vi "Finish.vi"   [LabVIEW 2014]
doc: "This VI is called just before exiting. It is expected to close I/O refnum, save collected data, etc."
uses:
  <vilib>/Rock Robotics/WPI/Joystick/WPI_JoystickGetSetRefNum.vi
  <vilib>/Rock Robotics/WPI/RobotDrive/WPI_RobotDriveGetSetRefNum.vi
  <vilib>/Rock Robotics/WPI/Compressor/WPI_CompressorGetSetRefNum.vi
types:
  T1 = typedef "WPI_MotorControlDeviceRef.ctl" = cluster{"DeviceStatus":errorcluster, "Type":T2, "PWM":cluster{"Controller":T3, "PWM Channel":T4, "DeadBand":T5}, "CAN":cluster{"Device Number":u8, "Control Mode":T6, "Semaphore":T7, "Max Vout":dbl, "TalonSRX Control Mode":T8}, "Invert":bool, "TransformRef":T9, "InvTransformRef":T9}
  T2 = typedef "WPI_MotorControlType.ctl" = enum16{"PWM", "CAN", "CANTalonSRX"}
  T3 = typedef "FPGA_TypedefDigitalModule.ctl" = enum16{"Controller 1"}
  T4 = typedef "FPGA_DIOPWMChannel.ctl" = enum8{"PWM 0", "PWM 1", "PWM 2", "PWM 3", "PWM 4", "PWM 5", "PWM 6", "PWM 7", "PWM 8", "PWM 9", "PWM MXP 0", "PWM MXP 1", "PWM MXP 2", "PWM MXP 3", "PWM MXP 4", "PWM MXP 5", "PWM MXP 6", "PWM MXP 7", "PWM MXP 8", "PWM MXP 9", "Invalid"}
  T5 = typedef "WPI_PWMDeadband.ctl" = cluster{"Name":string, "maxPositivePwm":i32, "minPositivePwm":i32, "centerPwm":i32, "maxNegativePwm":i32, "minNegativePwm":i32, "angularRange":u16}
  T6 = typedef "WPI_CANJaguar_ControlMode.ctl" = enum8{"Percent VBus", "Current", "Speed", "Position", "Voltage"}
  T7 = typedef "Semaphore RefNum" = refnum<k1>
  T8 = typedef "WPI_CANTalonSRX_APIControlMode.ctl" = enum8{"Percent VBus", "Speed", "Position", "Slave", "Unchanged / Invalid"}
  T9 = typedef "WPI_PWMTransform_ConPane.ctl" = refnum<vi>
  T10 = typedef "WPI_JoystickDevRef.ctl" = cluster{"Device":T11}
  T11 = typedef "WPI_JoystickDeviceEnum.ctl" = enum16{"USB 0", "USB 1", "USB 2", "USB 3", "USB 4", "USB 5"}
  T12 = typedef "WPI_RobotDriveDevRef.ctl" = cluster{"DevStatus":errorcluster, "Motors[]":T1[], "Square Inputs":bool, "Max Output":dbl}
  T13 = typedef "WPI_PotentiometerDevRef.ctl" = cluster{"DevStatus":errorcluster, "Controller":T14, "Analog Channel":T15, "Invert Output":bool}
  T14 = typedef "FPGA_TypedefAnalogModule.ctl" = enum16{"Controller 1"}
  T15 = typedef "FPGA_AIChannel.ctl" = enum8{"AI 0", "AI 1", "AI 2", "AI 3", "AI MXP 0", "AI MXP 1", "AI MXP 2", "AI MXP 3", "Invalid"}
  T16 = typedef "WPI_SolenoidDevRef.ctl" = cluster{"DevStatus":errorcluster, "Pneumatics Control Module":u8, "Forward Solenoid Channel":T17, "Reverse Solenoid Channel":T17}
  T17 = typedef "WPI_SolenoidChannel.ctl" = enum8{"Solenoid 0", "Solenoid 1", "Solenoid 2", "Solenoid 3", "Solenoid 4", "Solenoid 5", "Solenoid 6", "Solenoid 7", "Invalid"}
  T18 = typedef "WPI_SwitchDevRef.ctl" = cluster{"DevStatus":errorcluster, "DIO Channel":T19, "Controller":T3, "CntIndex":T20, "Normally Closed":bool}
  T19 = typedef "FPGA_DIOChannel.ctl" = enum8{"DIO 0", "DIO 1", "DIO 2", "DIO 3", "DIO 4", "DIO 5", "DIO 6", "DIO 7", "DIO 8", "DIO 9", "DIO MXP 0", "DIO MXP 1", "DIO MXP 2", "DIO MXP 3", "DIO MXP 4", "DIO MXP 5", "DIO MXP 6", "DIO MXP 7", "DIO MXP 8", "DIO MXP 9", "DIO MXP 10", "DIO MXP 11", "DIO MXP 12", "DIO MXP 13", "DIO MXP 14", "DIO MXP 15", "Invalid"}
  T20 = typedef "FPGA_CounterCtrSystemIndex.ctl" = enum8{"Ctr 0", "Ctr 1", "Ctr 2", "Ctr 3", "Ctr 4", "Ctr 5", "Ctr 6", "Ctr 7", "Invalid"}
  T21 = typedef "WPI_CompressorDevRef.ctl" = cluster{"DevStatus":errorcluster, "Pneumatics Control Module":u8}
  T22 = typedef "WPI_EncoderDevRef.ctl" = cluster{"DevStatus":errorcluster, "EncoderIndex":T23, "CounterIndex":T20, "DistancePerCount":dbl, "Decoding Type":T24}
  T23 = typedef "FPGA_EncoderIdx.ctl" = enum8{"Enc 0", "Enc 1", "Enc 2", "Enc 3", "Enc 4", "Enc 5", "Enc 6", "Enc 7", "Invalid"}
  T24 = typedef "WPI_EncoderType.ctl" = enum16{"1x", "2x", "4x"}
  T25 = typedef "WPI_GyroDevRef.ctl" = cluster{"DevStatus":errorcluster, "Analog Module":T14, "Analog Channel":T15, "Offset":dbl, "Gain (VoltsPerDegree/Second)":dbl}
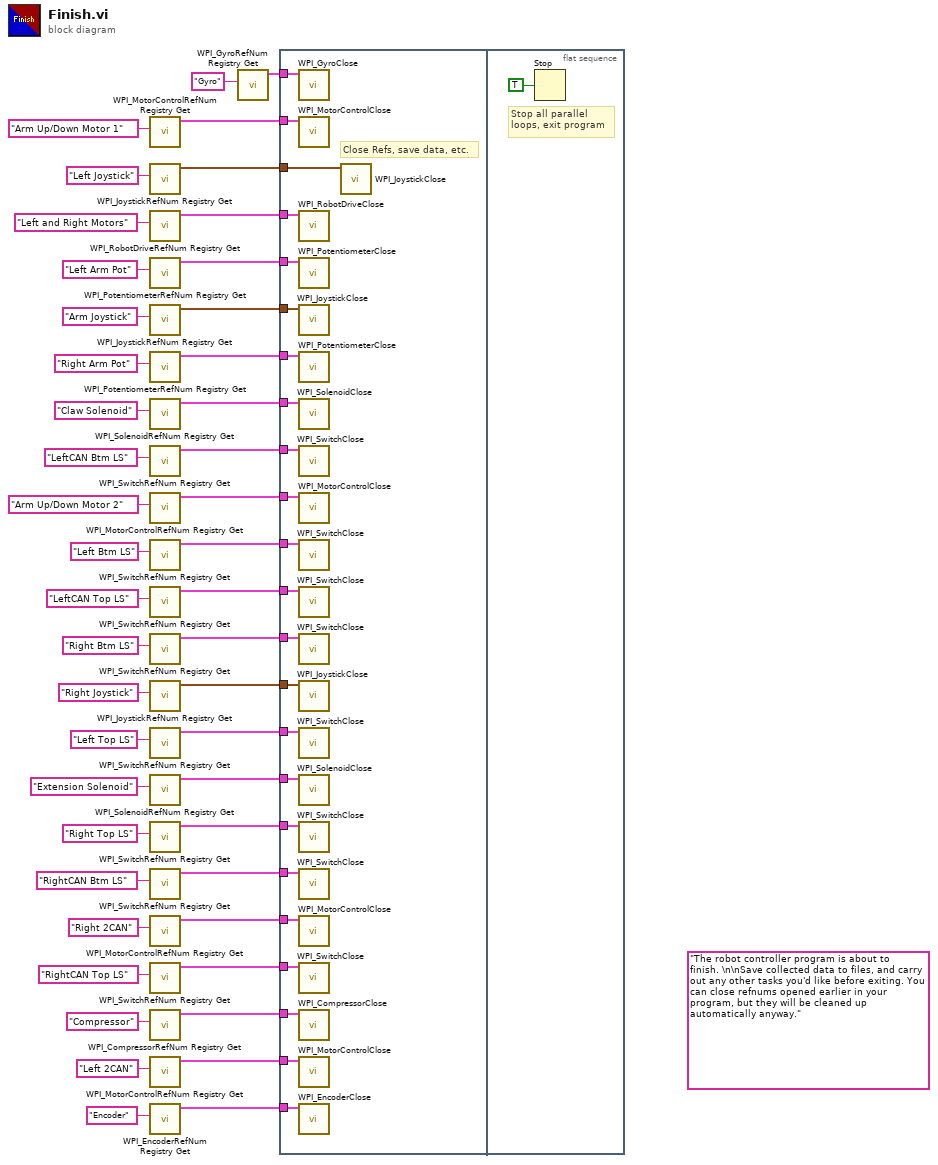
[diagram p0: block diagram]
diagram:
  (unwired) "The robot controller program is about to finish. \n\nSave collected data to files, and carry out any other tasks you'd like before exiting. You can close refnums opened earlier in your program, but they will be cleaned up automatically anyway."
  n1 = call <vilib>:"WPI_MotorControlRefNum Registry Get.vi"("refnum name"="Arm Up/Down Motor 1") -> ("MotorControlDevRef"=w33:T1)  [unwired: 9 in, 1 out]
  n2 = call <vilib>:"WPI_JoystickRefNum Registry Get.vi"("refnum name"="Left Joystick") -> ("JoystickDevRef"=w43:T10)  [unwired: 1 in, 9 out]
  n3 = call <vilib>:"WPI_RobotDriveRefNum Registry Get.vi"("refnum name"="Left and Right Motors") -> ("RobotDriveDevRef"=w44:T12)  [unwired: 1 in, 9 out]
  n4 = call <vilib>:"WPI_PotentiometerRefNum Registry Get.vi"("refnum name"="Left Arm Pot") -> ("PotDevRef"=w13:T13)  [unwired: 9 in, 1 out]
  n5 = call <vilib>:"WPI_JoystickRefNum Registry Get.vi"("refnum name"="Arm Joystick") -> ("JoystickDevRef"=w40:T10)  [unwired: 1 in, 9 out]
  n6 = call <vilib>:"WPI_PotentiometerRefNum Registry Get.vi"("refnum name"="Right Arm Pot") -> ("PotDevRef"=w12:T13)  [unwired: 9 in, 1 out]
  n7 = call <vilib>:"WPI_SolenoidRefNum Registry Get.vi"("refnum name"="Claw Solenoid") -> ("SolenoidDevRef"=w31:T16)  [unwired: 9 in, 1 out]
  n8 = call <vilib>:"WPI_SwitchRefNum Registry Get.vi"("refnum name"="LeftCAN Btm LS") -> ("SwitchDevRef"=w6:T18)  [unwired: 9 in, 1 out]
  n9 = call <vilib>:"WPI_MotorControlRefNum Registry Get.vi"("refnum name"="Arm Up/Down Motor 2") -> ("MotorControlDevRef"=w28:T1)  [unwired: 9 in, 1 out]
  n10 = call <vilib>:"WPI_SwitchRefNum Registry Get.vi"("refnum name"="Left Btm LS") -> ("SwitchDevRef"=w15:T18)  [unwired: 9 in, 1 out]
  n11 = call <vilib>:"WPI_SwitchRefNum Registry Get.vi"("refnum name"="LeftCAN Top LS") -> ("SwitchDevRef"=w5:T18)  [unwired: 9 in, 1 out]
  n12 = call <vilib>:"WPI_SwitchRefNum Registry Get.vi"("refnum name"="Right Btm LS") -> ("SwitchDevRef"=w16:T18)  [unwired: 9 in, 1 out]
  n13 = call <vilib>:"WPI_JoystickRefNum Registry Get.vi"("refnum name"="Right Joystick") -> ("JoystickDevRef"=w41:T10)  [unwired: 1 in, 9 out]
  n14 = call <vilib>:"WPI_SwitchRefNum Registry Get.vi"("refnum name"="Left Top LS") -> ("SwitchDevRef"=w17:T18)  [unwired: 9 in, 1 out]
  n15 = call <vilib>:"WPI_SolenoidRefNum Registry Get.vi"("refnum name"="Extension Solenoid") -> ("SolenoidDevRef"=w1:T16)  [unwired: 9 in, 1 out]
  n16 = call <vilib>:"WPI_SwitchRefNum Registry Get.vi"("refnum name"="Right Top LS") -> ("SwitchDevRef"=w18:T18)  [unwired: 9 in, 1 out]
  n17 = call <vilib>:"WPI_SwitchRefNum Registry Get.vi"("refnum name"="RightCAN Btm LS") -> ("SwitchDevRef"=w3:T18)  [unwired: 9 in, 1 out]
  n18 = call <vilib>:"WPI_MotorControlRefNum Registry Get.vi"("refnum name"="Right 2CAN") -> ("MotorControlDevRef"=w25:T1)  [unwired: 9 in, 1 out]
  n19 = call <vilib>:"WPI_SwitchRefNum Registry Get.vi"("refnum name"="RightCAN Top LS") -> ("SwitchDevRef"=w4:T18)  [unwired: 9 in, 1 out]
  n20 = call <vilib>:"WPI_CompressorRefNum Registry Get.vi"("refnum name"="Compressor") -> ("CompressorDevRef"=w29:T21)  [unwired: 9 in, 1 out]
  n21 = call <vilib>:"WPI_MotorControlRefNum Registry Get.vi"("refnum name"="Left 2CAN") -> ("MotorControlDevRef"=w24:T1)  [unwired: 9 in, 1 out]
  n22 = call <vilib>:"WPI_EncoderRefNum Registry Get.vi"("refnum name"="Encoder") -> ("EncoderDevRef"=w35:T22)  [unwired: 9 in, 1 out]
  n23 = call <vilib>:"WPI_GyroRefNum Registry Get.vi"("refnum name"="Gyro") -> ("GyroDevRef"=w37:T25)  [unwired: 9 in, 1 out]
  n24 = flat-sequence {
    tunnel: w44 -> [w69]
    tunnel: w43 -> [w68]
    tunnel: w41 -> [w67]
    tunnel: w40 -> [w66]
    tunnel: w37 -> [w65]
    tunnel: w35 -> [w64]
    tunnel: w33 -> [w63]
    tunnel: w31 -> [w62]
    tunnel: w29 -> [w61]
    tunnel: w28 -> [w60]
    tunnel: w24 -> [w58]
    tunnel: w25 -> [w59]
    tunnel: w18 -> [w57]
    tunnel: w17 -> [w56]
    tunnel: w16 -> [w55]
    tunnel: w15 -> [w54]
    tunnel: w13 -> [w53]
    tunnel: w12 -> [w52]
    tunnel: w6 -> [w51]
    tunnel: w5 -> [w50]
    tunnel: w4 -> [w49]
    tunnel: w3 -> [w48]
    tunnel: w1 -> [w47]
    frame #0 {
      # "Close Refs, save data, etc."
      n25 = call <vilib>:"WPI_GyroClose.vi"("GyroDevRef"=w65) -> ()  [unwired: 10 in, 1 out]
      n26 = call <vilib>:"WPI_MotorControlClose.vi"("MotorControlDevRef"=w63) -> ()  [unwired: 10 in, 1 out]
      n27 = call <vilib>:"WPI_RobotDriveClose.vi"("RobotDriveDevRef"=w69) -> ()  [unwired: 1 in, 10 out]
      n28 = call <vilib>:"WPI_PotentiometerClose.vi"("PotDevRef"=w53) -> ()  [unwired: 10 in, 1 out]
      n29 = call <vilib>:"WPI_JoystickClose.vi"("JoystickDevRef"=w66) -> ()  [unwired: 11 out]
      n30 = call <vilib>:"WPI_PotentiometerClose.vi"("PotDevRef"=w52) -> ()  [unwired: 10 in, 1 out]
      n31 = call <vilib>:"WPI_SolenoidClose.vi"("SolenoidDevRef"=w62) -> ()  [unwired: 10 in, 1 out]
      n32 = call <vilib>:"WPI_SwitchClose.vi"("SwitchDevRef"=w51) -> ()  [unwired: 10 in, 1 out]
      n33 = call <vilib>:"WPI_MotorControlClose.vi"("MotorControlDevRef"=w60) -> ()  [unwired: 10 in, 1 out]
      n34 = call <vilib>:"WPI_SwitchClose.vi"("SwitchDevRef"=w54) -> ()  [unwired: 10 in, 1 out]
      n35 = call <vilib>:"WPI_SwitchClose.vi"("SwitchDevRef"=w50) -> ()  [unwired: 10 in, 1 out]
      n36 = call <vilib>:"WPI_SwitchClose.vi"("SwitchDevRef"=w55) -> ()  [unwired: 10 in, 1 out]
      n37 = call <vilib>:"WPI_JoystickClose.vi"("JoystickDevRef"=w67) -> ()  [unwired: 11 out]
      n38 = call <vilib>:"WPI_SwitchClose.vi"("SwitchDevRef"=w56) -> ()  [unwired: 10 in, 1 out]
      n39 = call <vilib>:"WPI_SolenoidClose.vi"("SolenoidDevRef"=w47) -> ()  [unwired: 10 in, 1 out]
      n40 = call <vilib>:"WPI_SwitchClose.vi"("SwitchDevRef"=w57) -> ()  [unwired: 10 in, 1 out]
      n41 = call <vilib>:"WPI_SwitchClose.vi"("SwitchDevRef"=w48) -> ()  [unwired: 10 in, 1 out]
      n42 = call <vilib>:"WPI_MotorControlClose.vi"("MotorControlDevRef"=w59) -> ()  [unwired: 10 in, 1 out]
      n43 = call <vilib>:"WPI_SwitchClose.vi"("SwitchDevRef"=w49) -> ()  [unwired: 10 in, 1 out]
      n44 = call <vilib>:"WPI_CompressorClose.vi"("CompressorDevRef"=w61) -> ()  [unwired: 10 in, 1 out]
      n45 = call <vilib>:"WPI_MotorControlClose.vi"("MotorControlDevRef"=w58) -> ()  [unwired: 10 in, 1 out]
      n46 = call <vilib>:"WPI_EncoderClose.vi"("EncoderDevRef"=w64) -> ()  [unwired: 10 in, 1 out]
      n47 = call <vilib>:"WPI_JoystickClose.vi"("JoystickDevRef"=w68) -> ()  [unwired: 11 out]
    }
    frame #1 {
      # "Stop all parallel\nloops, exit program"
      n48 = Stop(stop? (T)=TRUE ("Quit")) -> ()
    }
  }
